vi "debugg.vi"() -> ()   [LabVIEW 2017]
panel:
  out "input-data-file-name":string
  in  "Array":string[](array[string])
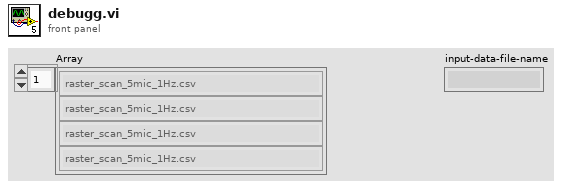
[diagram p1: front panel]
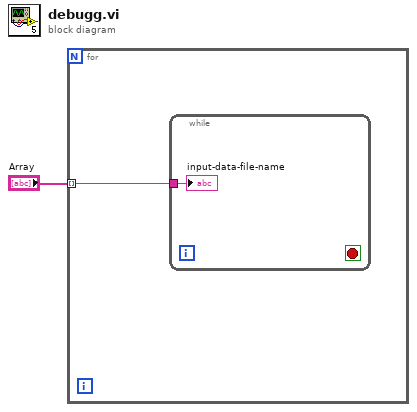
[diagram p0: block diagram]
diagram:
  n1 = for {
    tunnel: "Array" -> [w2] mode=indexing
    n2 = while {
      tunnel: w2 -> [w3]
      stop <- _ stop-if-true
      "input-data-file-name" <- w3
    }
  }
